vi "Write test data to nimbelink upload file Rev2.vi"(4 "Style":string, 6 "error in (no error)":errorcluster, 7 "imei":string, 8 "Meid":string, 9 "Serial Number":string) -> (0 "error out":errorcluster, 2 "PassFail":string, 3 "Write OK?":bool)   [LabVIEW 2013]
uses:
  Test Globals/Global 1.vi
  Main Support/Global 2.vi
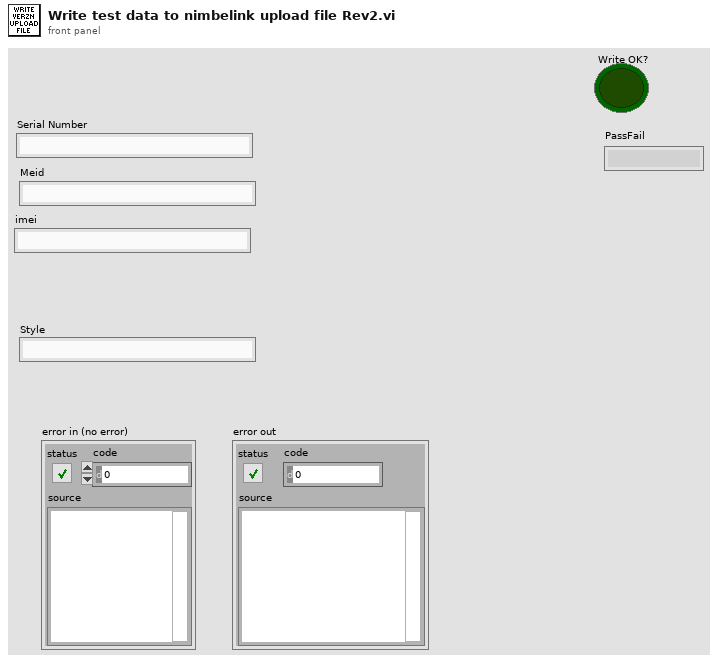
[diagram p1: front panel]
types:
  T1 = cluster{"Test folder":string, "Top level":string, "Main":string, "Test report":string, "Work order qty":string, "Work order meid":string, "Work order imei":string, "Master meid imei list":string, "Master test data":string, "ZPL label info":string, "Pictures":string, "Setup info":string, "Work order":string, "Tests folder":string, "Tests steps folder":string, "Config folder":string, "Verizon Upload file":string, "Job data file":string, "Station globals":string, "Post test info":string}
  T2 = enum16{"open", "replace", "create", "open or create", "replace or create", "replace or create with confirmation"}
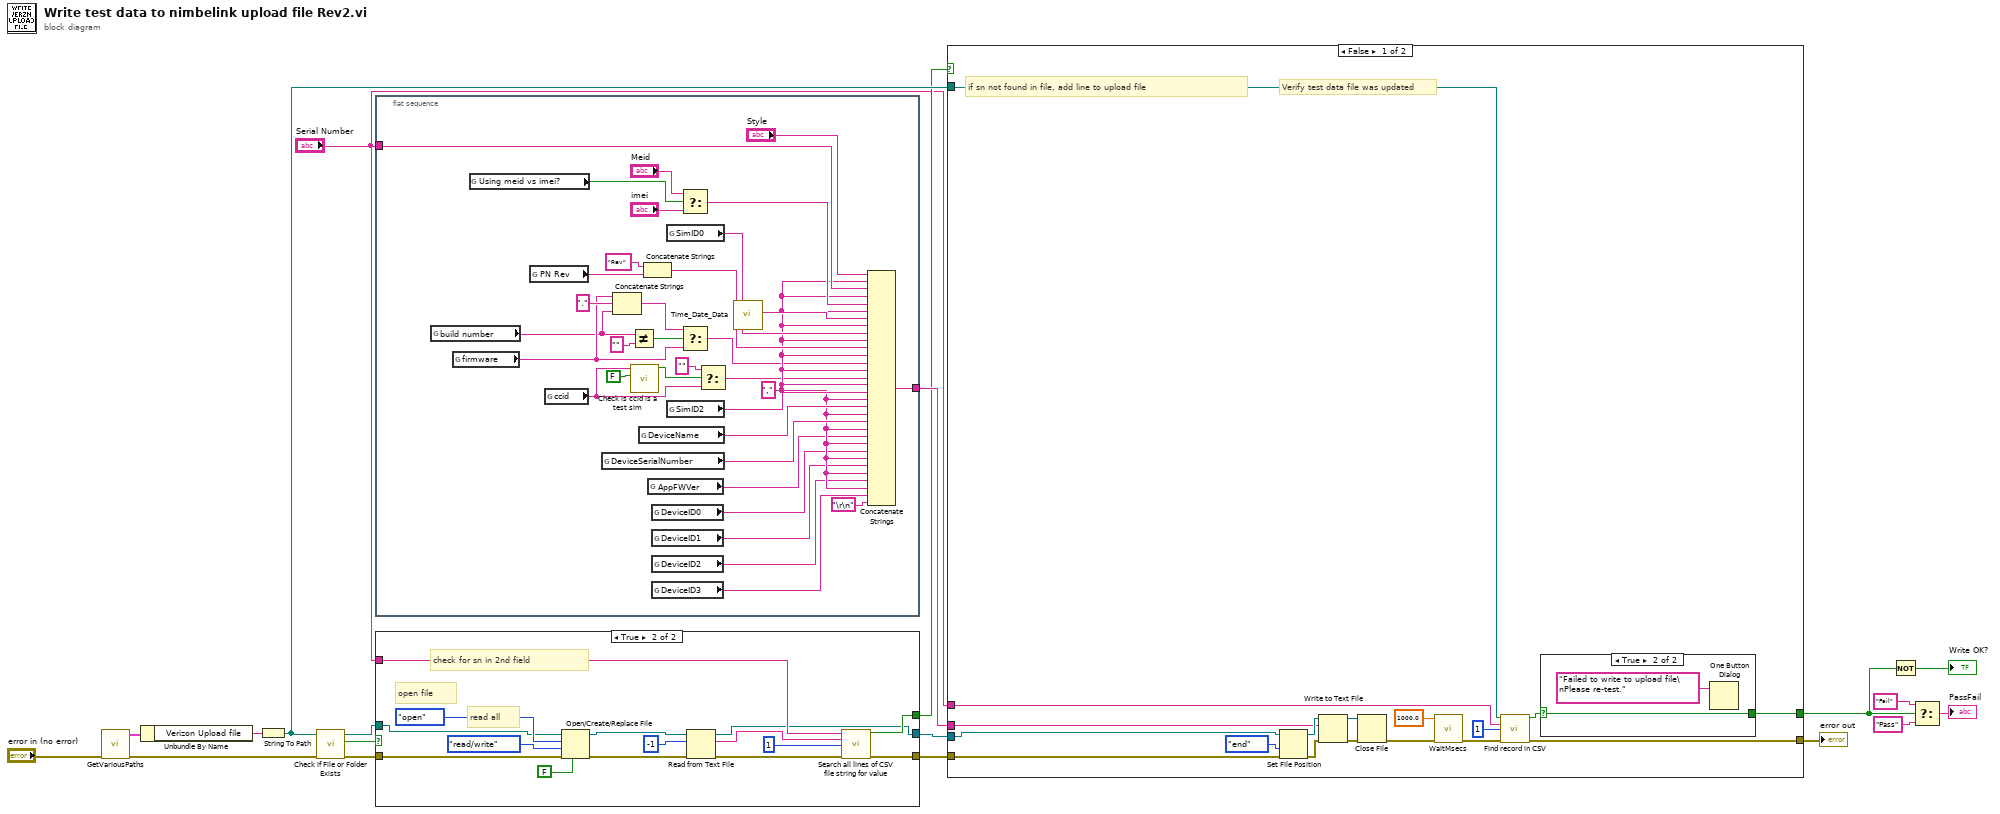
[diagram p0: block diagram]
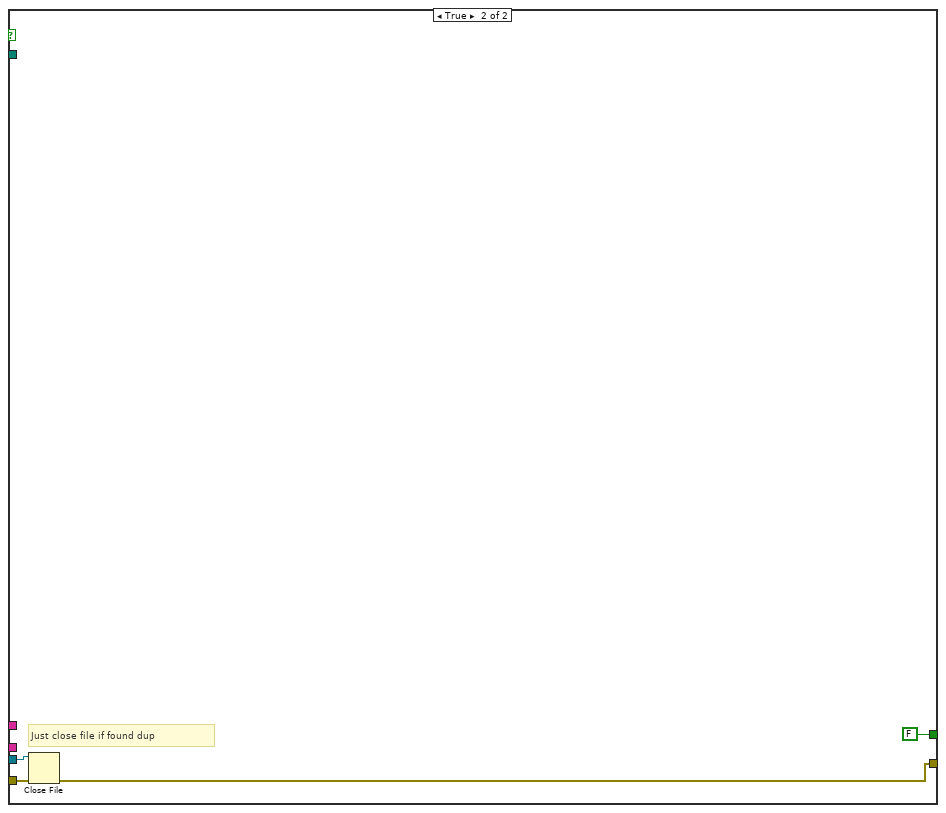
[diagram p3: hidden frame]
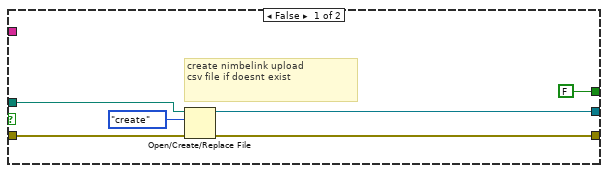
[diagram p4: hidden frame]
diagram:
  n1 = call "GetVariousPaths.vi"("error in (no error)"="error in (no error)") -> ("error out"=w15:errorcluster, "Built Paths"=w16:T1)  [unwired: 9 in]
  n2 = Unbundle By Name(w16) -> ("Verizon Upload file"=w17:string)
  n3 = String To Path(string=w17) -> (path=w14:path)
  n4 = call <vilib>:"Check if File or Folder Exists.vi"("error in (no error)"=w15, "path"=w14) -> ("error out"=w11:errorcluster, "file or folder exists?"=w13:bool, "dup path"=w12:path)  [unwired: 7 in]
  n5 = flat-sequence {
    tunnel: [w48] -> w7
    tunnel: "Serial Number" -> [w47]
    frame #0 {
      w37 = "," ("string")
      n6 = global read "Global 1.vi" "build number"() -> (w20:string)
      n7 = global read "Global 1.vi" "firmware"() -> (w22:string)
      n8 = global read "Global 1.vi" "Using meid vs imei?"() -> (w52:bool)
      n9 = global read "Global 2.vi" "PN Rev"() -> (w44:string)
      n10 = global read "Global 1.vi" "ccid"() -> (w27:string)
      n11 = global read "Global 1.vi" "DeviceSerialNumber"() -> (w39:string)
      n12 = Concatenate Strings(w22, "." ("string"), w20) -> (w23:string)
      n13 = Not Equal?(x=w20, y="") -> (x != y?=w25:bool)
      n14 = call "Check is ccid is a test sim.vi"("Use mem table? (y)"=FALSE ("Use mem table?"), "CCID"=w27) -> ("Result"=w30:bool)  [unwired: 6 in, 3 out]
      n15 = global read "Global 1.vi" "DeviceName"() -> (w40:string)
      n16 = Concatenate Strings("Rev" ("string"), w44) -> (w38:string)
      n17 = global read "Global 1.vi" "AppFWVer"() -> (w36:string)
      n18 = global read "Global 1.vi" "DeviceID0"() -> (w35:string)
      n19 = global read "Global 1.vi" "DeviceID1"() -> (w34:string)
      n20 = global read "Global 1.vi" "DeviceID2"() -> (w33:string)
      n21 = global read "Global 1.vi" "DeviceID3"() -> (w32:string)
      n22 = global read "Global 1.vi" "SimID0"() -> (w46:string)
      n23 = global read "Global 1.vi" "SimID2"() -> (w41:string)
      n24 = Select(t="Meid", s=w52, f="imei") -> (s? t:f=w49:string)
      n25 = Select(t=w23, s=w25, f=w22) -> (s? t:f=w21:string)
      n26 = Select(t="" ("f"), s=w30, f=w27) -> (s? t:f=w29:string)
      n27 = call "Time_Date_Data.vi"() -> ("UTC ISO 8601"=w42:string)  [unwired: 4 in, 7 out]
      n28 = Concatenate Strings("Style", w37, w47, w37, w49, w37, w42, w37, w46, w37, w38, w37, w21, w37, w29, w37, w41, w37, w40, w37, w39, w37, w36, w37, w35, w37, w34, w37, w33, w37, w32, "\r\n") -> (w48:string)
    }
  }
  n29 = case shown="True" w13 {
    tunnel: w12 -> [w58 w71]
    tunnel: w11 -> [w57 w70]
    tunnel: [w56 w62] -> w6
    tunnel: "Serial Number" -> [_ w64]
    tunnel: [FALSE ("Found value") w61] -> w5
    tunnel: [w55 w60] -> w4
    frame False {
      # "create nimbelink upload\ncsv file if doesnt exist"
      n30 = Open/Create/Replace File(file path (use dialog)=w58, error in=w57, operation (0:open)=T2."create") -> (refnum out=w55:refnum<file>, error out=w56:errorcluster)  [unwired: 3 in, 1 out]
    }
    frame True {
      # "check for sn in 2nd field"
      # "read all"
      # "open file"
      n31 = Open/Create/Replace File(file path (use dialog)=w71, error in=w70, operation (0:open)=T2."open", access (0:read/write)=enum16{"read/write", "read-only", "write-only"}."read/write", disable buffering (F)=FALSE) -> (refnum out=w68:refnum<file>, error out=w67:errorcluster)  [unwired: 1 in, 1 out]
      n32 = Read from Text File(file (use dialog)=w68, count=-1, error in=w67) -> (refnum out=w60:refnum<file>, text=w65:string, error out=w66:errorcluster)  [unwired: 1 in, 1 out]
      n33 = call "Search all lines of CSV file string for value.vi"("Compare value"=w64, "CSV file string"=w65, "CSV field (0-n)"=1, "error in"=w66) -> ("Found value"=w61:bool, "error out"=w62:errorcluster)  [unwired: 10 in]
    }
  }
  n34 = case shown="False" w5 {
    tunnel: [w77 w96] -> w2
    tunnel: w14 -> [w76 _]
    tunnel: w6 -> [w85 w97]
    tunnel: w7 -> [w88 _]
    tunnel: w4 -> [w84 w98]
    tunnel: [w78 FALSE] -> w3
    tunnel: "Serial Number" -> [w75 _]
    frame False {
      # "Verify test data file was updated"
      # "if sn not found in file, add line to upload file"
      n35 = Set File Position(refnum=w84, from (0:start)=enum16{"start", "end", "current"}."end", error in=w85) -> (refnum out=w89:refnum<file>, error out=w90:errorcluster)  [unwired: 1 in]
      n36 = Write to Text File(file (use dialog)=w89, text=w88, error in=w90) -> (refnum out=w86:refnum<file>, error out=w87:errorcluster)  [unwired: 1 in, 1 out]
      n37 = Close File(refnum=w86, error in=w87) -> (error out=w79:errorcluster)  [unwired: 1 out]
      n38 = call "WaitMsecs.vi"("error in (no error)"=w79, "Wait Msecs"=1000.0) -> ("error out"=w81:errorcluster)  [unwired: 9 in]
      n39 = call "Find record in CSV.vi"("CSV file"=w76, "Search key"=w75, "Search key column (0-n)"=u32 1, "error in"=w81) -> ("Record not found?"=w83:bool, "error out"=w77:errorcluster)  [unwired: 3 in, 7 out]
      n40 = case shown="True" w83 {
        selector: w83 -> [w92 w93]
        tunnel: [w92 w93] -> w78
        frame False {
        }
        frame True {
          n41 = One Button Dialog(message="Failed to write to upload file\nPlease re-test.") -> ()  [unwired: 1 in, 1 out]
        }
      }
    }
    frame True {
      # "Just close file if found dup"
      n42 = Close File(refnum=w98, error in=w97) -> (error out=w96:errorcluster)  [unwired: 1 out]
    }
  }
  "error out" <- w2
  n43 = Not(x=w3) -> (.not. x?=→"Write OK?":bool)
  n44 = Select(t="Fail" ("message"), s=w3, f="Pass" ("message")) -> (s? t:f=→"PassFail":string)
